vi "Convert_from_Pyhs.vi"(1 "group of DTC":dbl, 2 "type descriptor":T1) -> (0 "data out":u8[](array[numeric]))   [LabVIEW 2014]
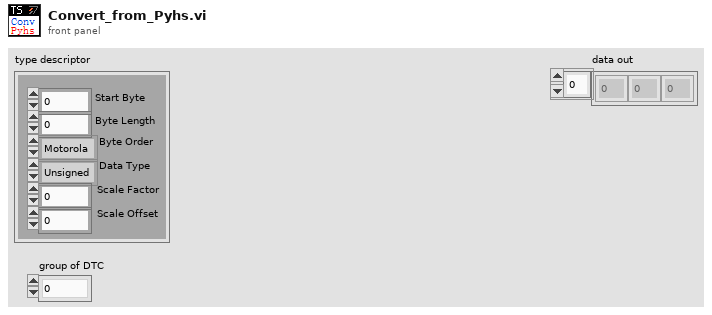
[diagram p1: front panel]
types:
  T1 = cluster{"Start Byte":i32, "Byte Length":i32, "Byte Order":enum16{"Motorola", "Intel"}, "Data Type":enum16{"Unsigned", "Signed", "Float"}, "Scale Factor":dbl, "Scale Offset":dbl}
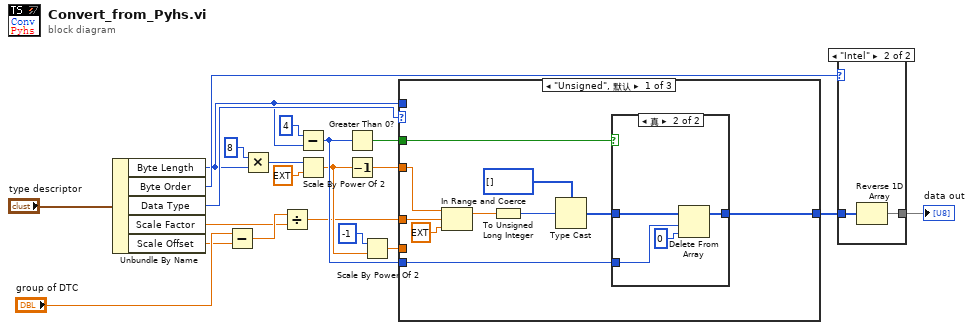
[diagram p0: block diagram]
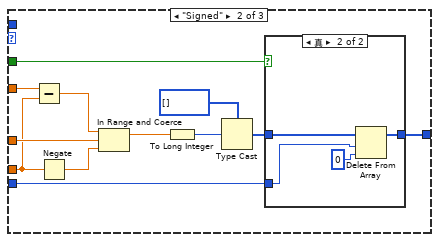
[diagram p3: hidden frame]
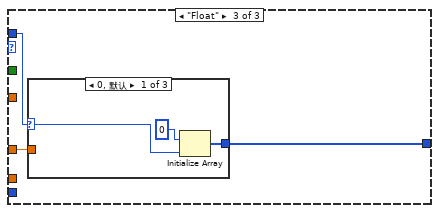
[diagram p5: hidden frame]
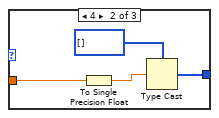
[diagram p6: hidden frame]
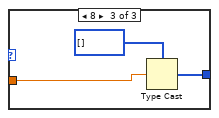
[diagram p7: hidden frame]
diagram:
  n1 = Unbundle By Name("type descriptor") -> ("Byte Length"=w6:i32, "Byte Order"=w11:enum16{"Motorola", "Intel"}, "Data Type"=w18:enum16{"Unsigned", "Signed", "Float"}, "Scale Factor"=w14:dbl, "Scale Offset"=w16:dbl)
  n2 = Subtract(x="group of DTC", y=w16) -> (x-y=w15:dbl)
  n3 = Multiply(x=8, y=w6) -> (x*y=w8:i32)
  n4 = Divide(x=w15, y=w14) -> (x/y=w3:dbl)
  n5 = Subtract(x=4, y=w6) -> (x-y=w19:i32)
  n6 = Scale By Power Of 2(n=w8, x=ext 1.0) -> (x*2^n=w5:ext)
  n7 = Greater Than 0?(x=w19) -> (x > 0?=w13:bool)
  n8 = Decrement(x=w5) -> (x-1=w2:ext)
  n9 = Scale By Power Of 2(n=-1, x=w5) -> (x*2^n=w1:ext)
  n10 = case shown="\"Unsigned\", 默认" w18 {
    tunnel: [w26 w44 w55] -> w12
    tunnel: w3 -> [w25 w41 w56]
    tunnel: w19 -> [w31 w48 _]
    tunnel: w13 -> [w27 w43 _]
    tunnel: w6 -> [_ _ w54]
    tunnel: w2 -> [w23 w39 _]
    tunnel: w1 -> [_ w37 _]
    frame "Unsigned", Default {
      n11 = In Range and Coerce(upper limit=w23, x=w25, lower limit=ext 0.0) -> (coerced(x)=w24:ext)  [unwired: 1 out]
      n12 = To Unsigned Long Integer(number=w24) -> (unsigned 32bit integer=w30:u32)
      n13 = Type Cast(type=u8[] [], x=w30) -> (*(type *) &x=w28:u8[])
      n14 = case shown="真" w27 {
        tunnel: w28 -> [w32 w36]
        tunnel: [w32 w35] -> w26
        tunnel: w31 -> [_ w34]
        frame False {
        }
        frame True {
          n15 = Delete From Array(array=w36, length=w34, index=0) -> (array with subset deleted=w35:u8[])  [unwired: 1 out]
        }
      }
    }
    frame "Signed" {
      n16 = Subtract(x=w39, y=w37) -> (x-y=w40:ext)
      n17 = Negate(x=w37) -> (-x=w38:ext)
      n18 = In Range and Coerce(upper limit=w40, x=w41, lower limit=w38) -> (coerced(x)=w42:ext)  [unwired: 1 out]
      n19 = To Long Integer(number=w42) -> (32bit integer=w47:i32)
      n20 = Type Cast(type=u8[] [], x=w47) -> (*(type *) &x=w45:u8[])
      n21 = case shown="真" w43 {
        tunnel: w45 -> [w49 w52]
        tunnel: [w49 w51] -> w44
        tunnel: w48 -> [_ w53]
        frame False {
        }
        frame True {
          n22 = Delete From Array(array=w52, length=w53, index=0) -> (array with subset deleted=w51:u8[])  [unwired: 1 out]
        }
      }
    }
    frame "Float" {
      n23 = case shown="0, 默认" w54 {
        selector: w54 -> [w57 _ _]
        tunnel: w56 -> [_ w62 w64]
        tunnel: [w59 w63 w66] -> w55
        frame 0, Default {
          n24 = Initialize Array(u8 0 ("element"), w57) -> (w59:u8[])
        }
        frame 4 {
          n25 = To Single Precision Float(number=w62) -> (single precision float=w61:sgl)
          n26 = Type Cast(type=u8[] [], x=w61) -> (*(type *) &x=w63:u8[])
        }
        frame 8 {
          n27 = Type Cast(type=u8[] [], x=w64) -> (*(type *) &x=w66:u8[])
        }
      }
    }
  }
  n28 = case shown="\"Intel\"" w11 {
    tunnel: [w67 w69] -> w10
    tunnel: w12 -> [w67 w68]
    frame "Motorola", Default {
    }
    frame "Intel" {
      n29 = Reverse 1D Array(array=w68) -> (reversed array=w69:u8[])
    }
  }
  "data out" <- w10
